vi "BaseProvider_ConfigurationMemory.vi"(1 "WireConfiguration":T2={"Edge thickness"=1, "Edge color"=5667411, "Center thickness"=1, "Center pattern"=enum."Solid", "CenterColor1"=9740924, "CenterColor2"=8694662, "Tunnels and terminals colors"=131187}, 2 "Icon":string="bluefull.png", 4 "Filter_Icons":bool, 5 "error in (no error)":errorcluster, 6 "Action":enum16{"Read", "Load", "Save", "Set"}(ring), 7 "PatternIn":T1 items=["4x4x4", "5x6x5", "6x8x6"]) -> (12 "ClassItemIconGroup":string[](array[string]), 13 "PatternOut":T1 items=["4x4x4", "5x6x5", "6x8x6"], 15 "WireConfigurationOut":T2={"Edge thickness"=1, "Edge color"=5667411, "Center thickness"=1, "Center pattern"=enum."Solid", "CenterColor1"=9740924, "CenterColor2"=8694662, "Tunnels and terminals colors"=131187}, 16 "IconOut":string="bluefull.png", 17 "ClassItemIconPaths":path[](array[path]), 18 "ClassItemIconNames":string[](array[string]), 19 "error out":errorcluster)   [LabVIEW 2014]
uses:
  <resource>/Framework/Providers/Open_GDS/SubVIs/GOOP_WireConfigurationType.ctl
  <resource>/Framework/Providers/Open_GDS/SubVIs/GOOP_WirePattern.ctl
  <resource>/Framework/Providers/Open_GDS/ClassProviders/Common/ScriptingFunctions/Scripting_ConnectorPanePatternType.ctl
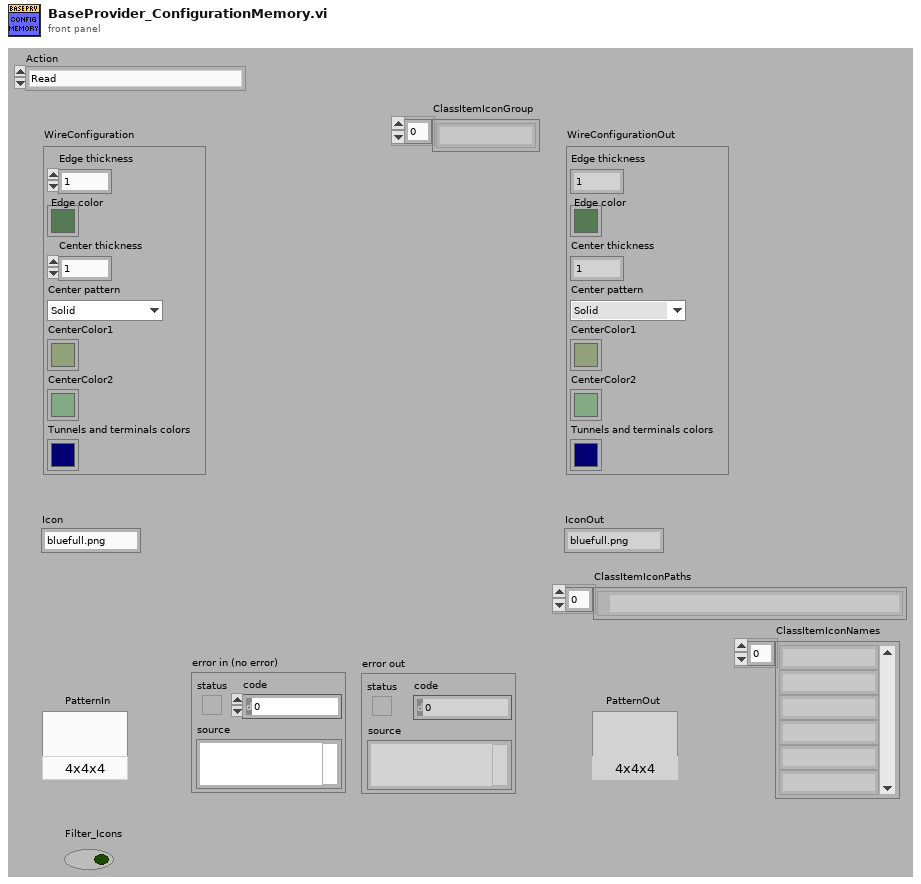
[diagram p1: front panel]
types:
  T1 = typedef "Scripting_ConnectorPanePatternType.ctl" = u16
  T2 = typedef "GOOP_WireConfigurationType.ctl" = cluster{"Edge thickness":i32, "Edge color":u32, "Center thickness":i32, "Center pattern":T3, "CenterColor1":u32, "CenterColor2":u32, "Tunnels and terminals colors":u32}
  T3 = typedef "GOOP_WirePattern.ctl" = enum16{"Solid", "Large dash", "Small dash"}
  T4 = cluster{"WireConfiguration":T2, "Icon":string, "Pattern":T1}
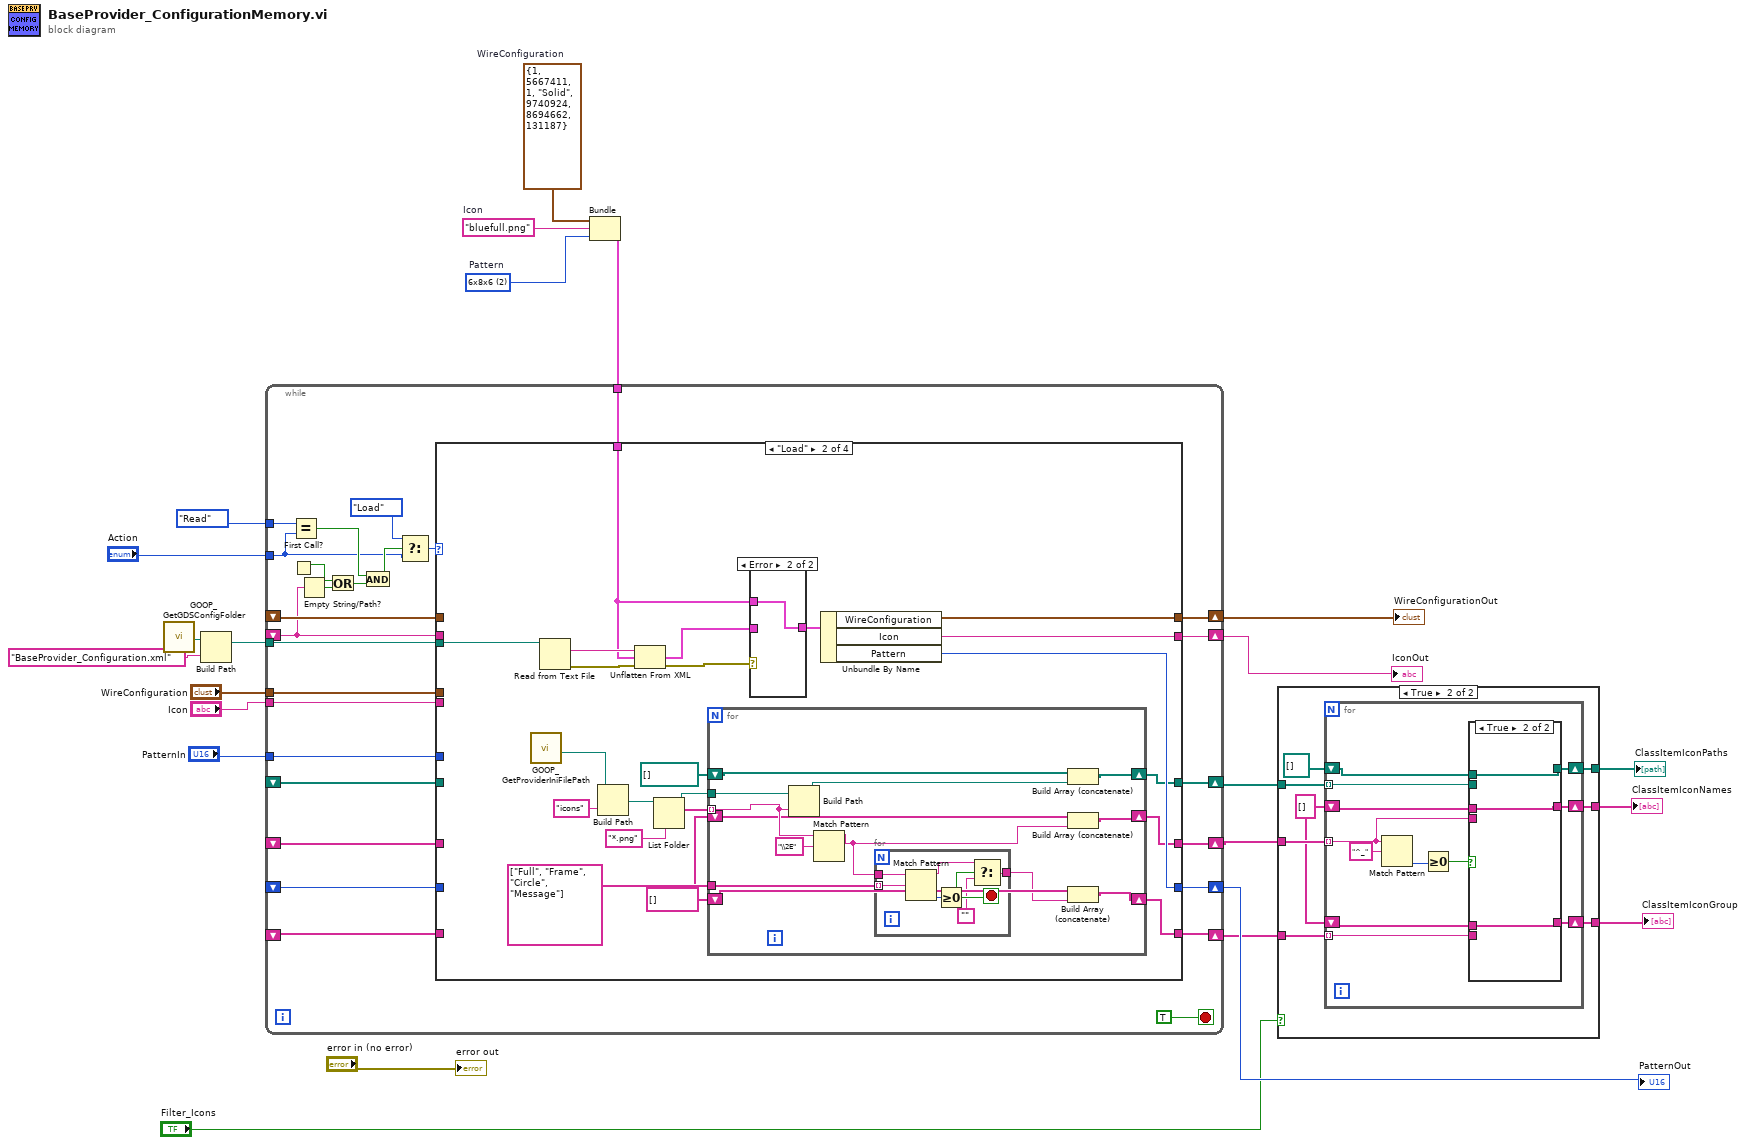
[diagram p0: block diagram]
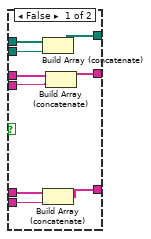
[diagram p3: hidden frame]
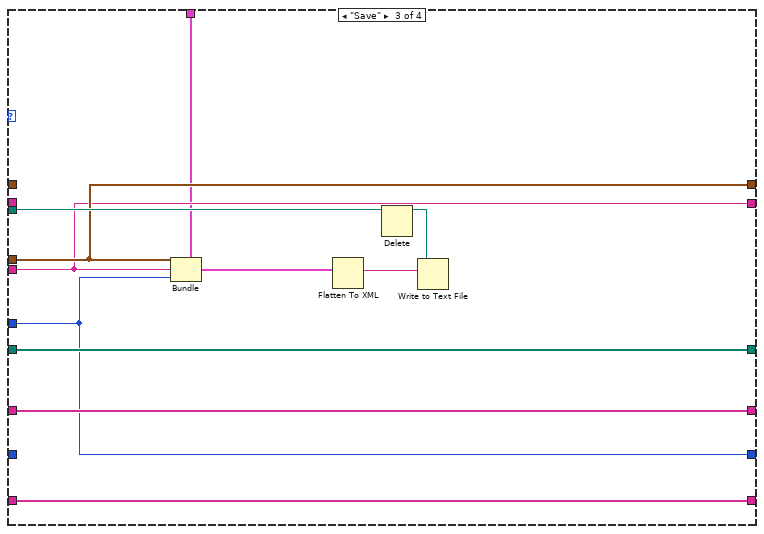
[diagram p6: hidden frame]
diagram:
  w12 = T1 2 items=["4x4x4", "5x6x5", "6x8x6"]  # Pattern
  w19 = "bluefull.png"  # Icon
  w20 = T2 {"Edge thickness"=1, "Edge color"=5667411, "Center thickness"=1, "Center pattern"=enum."Solid", "CenterColor1"=9740924, "CenterColor2"=8694662, "Tunnels and terminals colors"=131187}  # WireConfiguration
  n1 = call <resource>:"GOOP_GetGDSConfigFolder.vi"() -> ("GDSFolderPath"=w22:path)
  n2 = Build Path(base path=w22, name or relative path="BaseProvider_Configuration.xml") -> (appended path=w21:path)
  n3 = Bundle("WireConfiguration"=w20, "Icon"=w19, "Pattern"=w12) -> (w18:T4)  [unwired: 1 in]
  n4 = while {
    tunnel: "Action" -> [w26]
    tunnel: w21 -> [w50]
    tunnel: w18 -> [w49]
    shift-right: [w47] -> w17
    shift-left: _ -> [w45]
    shift-right: [w46] -> w16
    shift-left: _ -> [w33]
    shift-right: [w44] -> w8
    shift-left: _ -> [w43]
    shift-right: [w42] -> w9
    shift-left: _ -> [w41]
    tunnel: "WireConfiguration" -> [w40]
    tunnel: "Icon" -> [w39]
    shift-right: [w37] -> w10
    shift-left: _ -> [w36]
    tunnel: "PatternIn" -> [w38]
    shift-right: [w35] -> w7
    shift-left: _ -> [w34]
    tunnel: enum16{"Read", "Load", "Save", "Set"}."Read" ("t") -> [w32]
    stop <- TRUE stop-if-true
    n5 = First Call?() -> (First Call?: T/F=w30:bool)
    n6 = Equal?(x=w32, y=w26) -> (x = y?=w28:bool)
    n7 = Empty String/Path?(string/path=w33) -> (empty?=w31:bool)
    n8 = Or(x=w30, y=w31) -> (x .or. y?=w29:bool)
    n9 = And(x=w28, y=w29) -> (x .and. y?=w27:bool)
    n10 = Select(t=enum16{"Read", "Load", "Save", "Set"}."Load", s=w27, f=w26) -> (s? t:f=w25:enum16{"Read", "Load", "Save", "Set"})
    n11 = case shown="\"Load\"" w25 {
      tunnel: w50 -> [_ w73 w107 _]
      tunnel: w49 -> [_ w72 w103 _]
      tunnel: [w56 w71 w105 w115] -> w47
      tunnel: [w55 w70 w104 w114] -> w46
      tunnel: w45 -> [w56 _ _ _]
      tunnel: w33 -> [w55 _ _ _]
      tunnel: [w54 w60 w111 w117] -> w44
      tunnel: w43 -> [w54 _ w111 w117]
      tunnel: [w53 w57 w108 w116] -> w42
      tunnel: w41 -> [w53 _ w108 w116]
      tunnel: w40 -> [_ _ w105 w115]
      tunnel: w39 -> [_ _ w104 w114]
      tunnel: w38 -> [_ _ w102 w113]
      tunnel: [w52 w63 w102 w113] -> w37
      tunnel: w36 -> [w52 _ _ _]
      tunnel: [w51 w58 w101 w112] -> w35
      tunnel: w34 -> [w51 _ w101 w112]
      frame "Read", Default {
      }
      frame "Load" {
        w59 = string[] []
        n12 = call <resource>:"GOOP_GetProviderIniFilePath.vi"() -> ("ProviderMainFolder"=w66:path)  [unwired: 10 in, 1 out]
        n13 = Read from Text File(file (use dialog)=w73) -> (text=w74:string, error out=w75:errorcluster)  [unwired: 3 in, 2 out]
        n14 = Build Path(base path=w66, name or relative path="icons") -> (appended path=w68:path)
        n15 = Unflatten From XML(xml string=w74, type=w72, error in (no error)=w75) -> (value=w77:T4, error out=w76:errorcluster)
        n16 = List Folder(path=w68, pattern="*.png") -> (path out=w64:path, filenames=w65:string[])  [unwired: 2 in, 2 out]
        n17 = for {
          tunnel: w65 -> [w88] mode=indexing
          tunnel: w64 -> [w91]
          tunnel: string[] ["Full", "Frame", "Circle", "Message"] -> [w89]
          shift-right: [w86] -> w60
          shift-left: path[] [] -> [w85]
          shift-right: [w84] -> w57
          shift-left: w59 -> [w81]
          shift-right: [w83] -> w58
          shift-left: w59 -> [w82]
          n18 = Build Path(base path=w91, name or relative path=w88) -> (appended path=w87:path)
          n19 = Match Pattern(string=w88, regular expression="\\2E") -> (before substring=w80:string)  [unwired: 1 in, 3 out]
          n20 = for {
            tunnel: w80 -> [w98]
            tunnel: w89 -> [w97] mode=indexing
            tunnel: [w93] -> w79
            stop <- w95 stop-if-true
            n21 = Match Pattern(string=w98, regular expression=w97) -> (before substring=w94:string, offset past match=w96:i32)  [unwired: 1 in, 2 out]
            n22 = Greater Or Equal To 0?(x=w96) -> (x >= 0?=w95:bool)
            n23 = Select(t=w94, s=w95, f="") -> (s? t:f=w93:string)
          }
          n24 = Build Array (concatenate)(w85, w87) -> (w86:path[])
          n25 = Build Array (concatenate)(w81, w80) -> (w84:string[])
          n26 = Build Array (concatenate)(w82, w79) -> (w83:string[])
        }
        n27 = case shown="Error" w76 {
          tunnel: w77 -> [w99 _]
          tunnel: [w99 w100] -> w78
          tunnel: w72 -> [_ w100]
          frame No Error {
          }
          frame Error {
          }
        }
        n28 = Unbundle By Name(w78) -> ("WireConfiguration"=w71:T2, "Icon"=w70:string, "Pattern"=w63:T1)
      }
      frame "Save" {
        n29 = Bundle(cluster=w103, "WireConfiguration"=w105, "Icon"=w104, "Pattern"=w102) -> (w106:T4)
        n30 = Flatten To XML(anything=w106) -> (xml string=w109:string)
        n31 = Delete(path (use dialog)=w107) -> (deleted path=w110:path)  [unwired: 4 in, 2 out]
        n32 = Write to Text File(file (use dialog)=w110, text=w109) -> ()  [unwired: 2 in, 3 out]
      }
      frame "Set" {
      }
    }
  }
  "WireConfigurationOut" <- w17
  "IconOut" <- w16
  "PatternOut" <- w10
  n33 = case shown="True" "Filter_Icons" {
    tunnel: w9 -> [w119 w128]
    tunnel: w8 -> [w120 w127]
    tunnel: w7 -> [w118 w126]
    tunnel: [w120 w123] -> w6
    tunnel: [w119 w122] -> w5
    tunnel: [w118 w121] -> w4
    frame False {
    }
    frame True {
      w124 = string[] []
      n34 = for {
        tunnel: w128 -> [w135] mode=indexing
        tunnel: w127 -> [w137] mode=indexing
        tunnel: w126 -> [w136] mode=indexing
        shift-right: [w130] -> w123
        shift-left: path[] [] -> [w129]
        shift-right: [w131] -> w122
        shift-left: w124 -> [w132]
        shift-right: [w134] -> w121
        shift-left: w124 -> [w133]
        n35 = Match Pattern(string=w135, regular expression="^_") -> (offset past match=w139:i32)  [unwired: 1 in, 3 out]
        n36 = Greater Or Equal To 0?(x=w139) -> (x >= 0?=w138:bool)
        n37 = case shown="True" w138 {
          tunnel: w137 -> [w149 _]
          tunnel: w136 -> [w147 _]
          tunnel: w135 -> [w148 _]
          tunnel: [w146 w150] -> w134
          tunnel: w133 -> [w145 w150]
          tunnel: w132 -> [w144 w151]
          tunnel: [w143 w151] -> w131
          tunnel: [w142 w152] -> w130
          tunnel: w129 -> [w141 w152]
          frame False {
            n38 = Build Array (concatenate)(w141, w149) -> (w142:path[])
            n39 = Build Array (concatenate)(w145, w147) -> (w146:string[])
            n40 = Build Array (concatenate)(w144, w148) -> (w143:string[])
          }
          frame True {
          }
        }
      }
    }
  }
  "ClassItemIconPaths" <- w6
  "ClassItemIconNames" <- w5
  "ClassItemIconGroup" <- w4
  "error out" <- "error in (no error)"
